vi "Vision info.vi"() -> ()   [LabVIEW 2018]
panel:
  out "Type taken":enum16{"Z", "I", "O", "S", "L", "J", "T", "N"}(ring)
  in  "frames":i32
  out "pice found":bool
  out "angel":dbl
  out "Type":enum16{"Z", "I", "O", "S", "L", "J", "T", "N"}(ring)
  out "dy":dbl
  out "dx":dbl
  out "pice found 3":bool
  out "angel 3":dbl
  out "Type  3":enum16{"Z", "I", "O", "S", "L", "J", "T", "N"}(ring)
  out "dy 3":dbl
  out "dx 3":dbl
  out "pice found 2":bool
  out "angel 2":dbl
  out "Type  2":enum16{"Z", "I", "O", "S", "L", "J", "T", "N"}(ring)
  out "dy 2":dbl
  out "dx 2":dbl
  out "pice found 1":bool
  out "angel 1":dbl
  out "Type  1":enum16{"Z", "I", "O", "S", "L", "J", "T", "N"}(ring)
  out "dy 1":dbl
  out "dx 1":dbl
  out "pice found 0":bool
  out "angel 0":dbl
  out "Type 0":enum16{"Z", "I", "O", "S", "L", "J", "T", "N"}(ring)
  out "dy 0":dbl
  out "dx 0":dbl
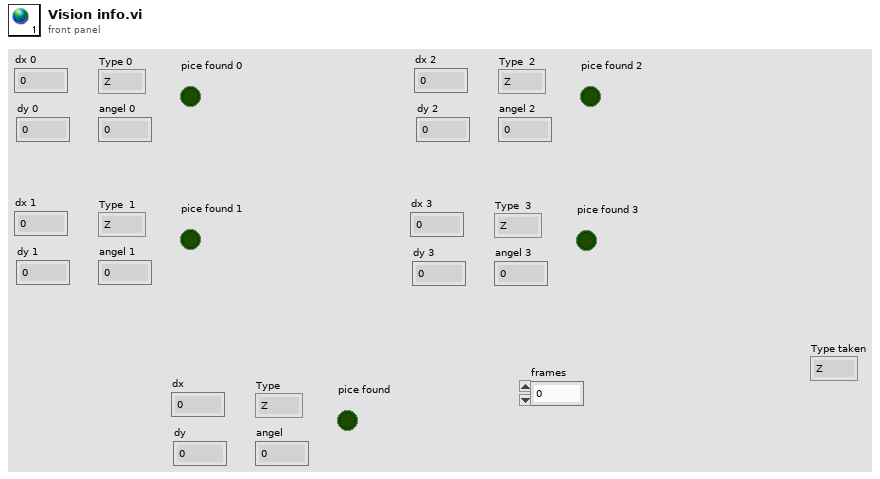
[diagram p1: front panel]
diagram:
